vi "simulate encoder.vi"(8 "error in (no error)":errorcluster, 11 "channel":u16) -> (0 "error out":errorcluster)   [LabVIEW 2015, in "SCANalone4x64.lvlib"]
doc: "__declspec(dllimport) void __stdcall simulate_encoder(unsigned short channel);"
uses:
  <userlib>/SCANalone4x64/SCANalone4x64.lvlib
  <userlib>/SCANalone4x64/SCANalone4x64.dll
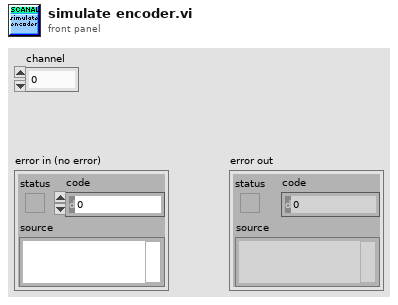
[diagram p1: front panel]
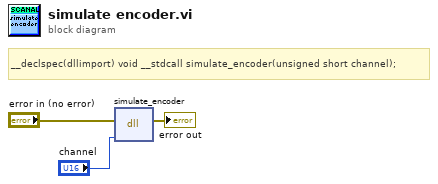
[diagram p0: block diagram]
diagram:
  # "__declspec(dllimport) void __stdcall simulate_encoder(unsigned short channel);"
  n1 = dll-call lib="C:/Program Files/National Instruments/LabVIEW 2015/user.lib/SCANalone4x64/SCANalone4x64.*" fn="simulate_encoder"(error in="error in (no error)", "channel"="channel") -> (error out=→"error out":errorcluster)  [unwired: 4 in, 1 out]
